vi "Find XML Config Path.vi"(10 "Files Generated by Build":path[](array[path])) -> (1 "Found ?":bool, 2 "XML Config Path":path)   [LabVIEW 2019, in "LVLIBP CD XML Updater.lvlib"]
uses:
  LVLIBP CD XML Updater.lvlib
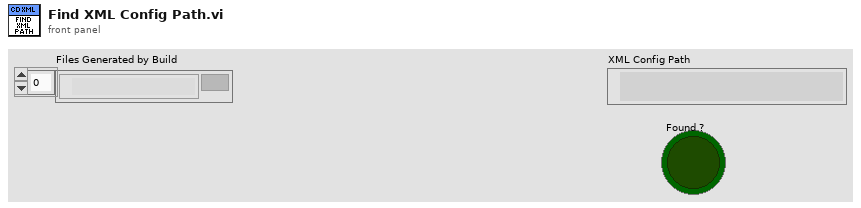
[diagram p1: front panel]
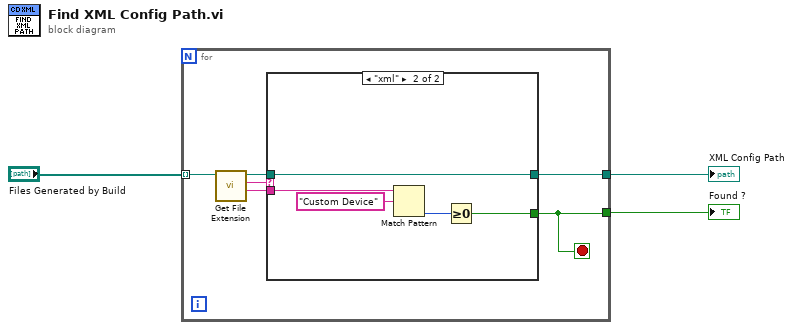
[diagram p0: block diagram]
diagram:
  n1 = for {
    tunnel: "Files Generated by Build" -> [w9] mode=indexing
    tunnel: [w5] -> w1
    tunnel: [w4] -> w2
    stop <- w5 stop-if-true
    n2 = call <vilib>:"Get File Extension.vi"("file"=w9) -> ("filename without extension"=w7:string, "lowercase file extension"=w8:string, "dup file"=w6:path)  [unwired: 6 in, 2 out]
    n3 = case shown="\"xml\"" w8 {
      tunnel: w7 -> [_ w14]
      tunnel: w6 -> [_ w11]
      tunnel: [_ w12] -> w5
      tunnel: [_ w11] -> w4
      frame "None", Default {
      }
      frame "xml" {
        n4 = Match Pattern(string=w14, regular expression="Custom Device") -> (offset past match=w13:i32)  [unwired: 1 in, 3 out]
        n5 = Greater Or Equal To 0?(x=w13) -> (x >= 0?=w12:bool)
      }
    }
  }
  "XML Config Path" <- w2
  "Found ?" <- w1
